vi "LabviewClaDInterface.vi"() -> ()   [LabVIEW 2016]
uses:
  <userlib>/ROS for LabVIEW Software/ROS/Code/SubVIs/_ROSControl.ctl
  <userlib>/ROS for LabVIEW Software/ROS/Code/SubVIs/_ROSDirection.ctl
  <userlib>/ROS for LabVIEW Software/ROS/Code/Console/Servers/ServerSubs/TopicDef.ctl
  <userlib>/ROS for LabVIEW Software/ROS/MessageBuilding/std_msgs/subs/stringScalar.vi
  <userlib>/ROS for LabVIEW Software/ROS/MessageParsing/std_msgs/subs/parse_string_scalar.vi
panel:
  out "Odom Error Out":errorcluster
  out "Scan Error Out":errorcluster
  in  "Stop Subscribing":bool
  out "Husky Pose Plot":cluster{"X":dbl, "Y":dbl}[](graph)=[{"X"=2.1588546690121686, "Y"=0.6824320147682317}]
  out "Laser Scan Plot (in Husky Frame)":cluster{dbl[], dbl[]}(graph)
  out "Husky EKF Odometry":T1={"PoseCovariance"={"Pose"={"Position\n(xyz)"={"x"=2.1588546690121686, "y"=0.6824320147682317, "z"=0.0}, "Orientation\n(Quaternions)"={"x"=0.0, "y"=0.0, "z"=-0.6154075833582808, "w"=0.7882090499005455}}, "Covariance[1,1]"=150.49515067805697}}
  out "2D Pose":cluster{"x":dbl, "y":dbl}={"x"=2.1588546690121686, "y"=0.6824320147682317}
  in  "Update Time (ms)":u32=300
  in  "Clear Plot":bool
  out "Scan Details":T2={"Min. Angle (rad)"=-2.3561899662017822, "Max. Angle (rad)"=2.3561899662017822, "Angle Incr. (rad)"=0.006554075051099062, "Time Inc. (s)"=0.0, "Scan Time (s)"=0.0, "Min. Range (m)"=0.10000000149011612, "Max. Range (m)"=1.0089348943138683e-42}
  in  "Max Odom Pts":dbl=500.0
  out "Robot Velocity":dbl(knob) scale=0.0..10.0
  out "ROS velocity_labview":T3={"topic port"=0, "Node"="", "topic"="", "type"="", "node port"=0, "error "={"status"=FALSE, "code"=0, "source"=""}, "Direction"=enum."Node", "Update (ms)"=1, "FIFO size"=1}
  out "ROS Manuel process":T3={"topic port"=0, "Node"="", "topic"="", "type"="", "node port"=0, "error "={"status"=FALSE, "code"=0, "source"=""}, "Direction"=enum."Node", "Update (ms)"=1, "FIFO size"=1}
  in  "velocity Process Stop":bool
  out "XY Graph":cluster{"X":dbl, "Y":dbl}[](graph)
  in  "Manuel Process Stop":bool
  in  "Message":string
  in  "Autonomous Process Stop":bool
  in  "Right":bool
  in  "Left":bool
  in  "Down":bool
  in  "Up":bool
  in  "Process Stop":bool
  in  "Home":bool
  out "Table  8":bool
  out "Table  7":bool
  out "Table  6":bool
  in  "OK Button":bool
  in  "table 8":bool
  in  "table 7":bool
  out "ROS Autonomous control":T3={"topic port"=0, "Node"="", "topic"="", "type"="", "node port"=0, "error "={"status"=FALSE, "code"=0, "source"=""}, "Direction"=enum."Node", "Update (ms)"=1, "FIFO size"=1}
  in  "table 6":bool
  in  "table 5":bool
  in  "table 4":bool
  in  "table 3":bool
  in  "table2":bool
  in  "table 1":bool
  out "ROS Autonomous indicator Tables":T3={"topic port"=0, "Node"="", "topic"="", "type"="", "node port"=0, "error "={"status"=FALSE, "code"=0, "source"=""}, "Direction"=enum."Node", "Update (ms)"=1, "FIFO size"=1}
  out "Table  5":bool
  out "Table  4":bool
  out "Table  3":bool
  out "Table  2":bool
  out "Table 1":bool
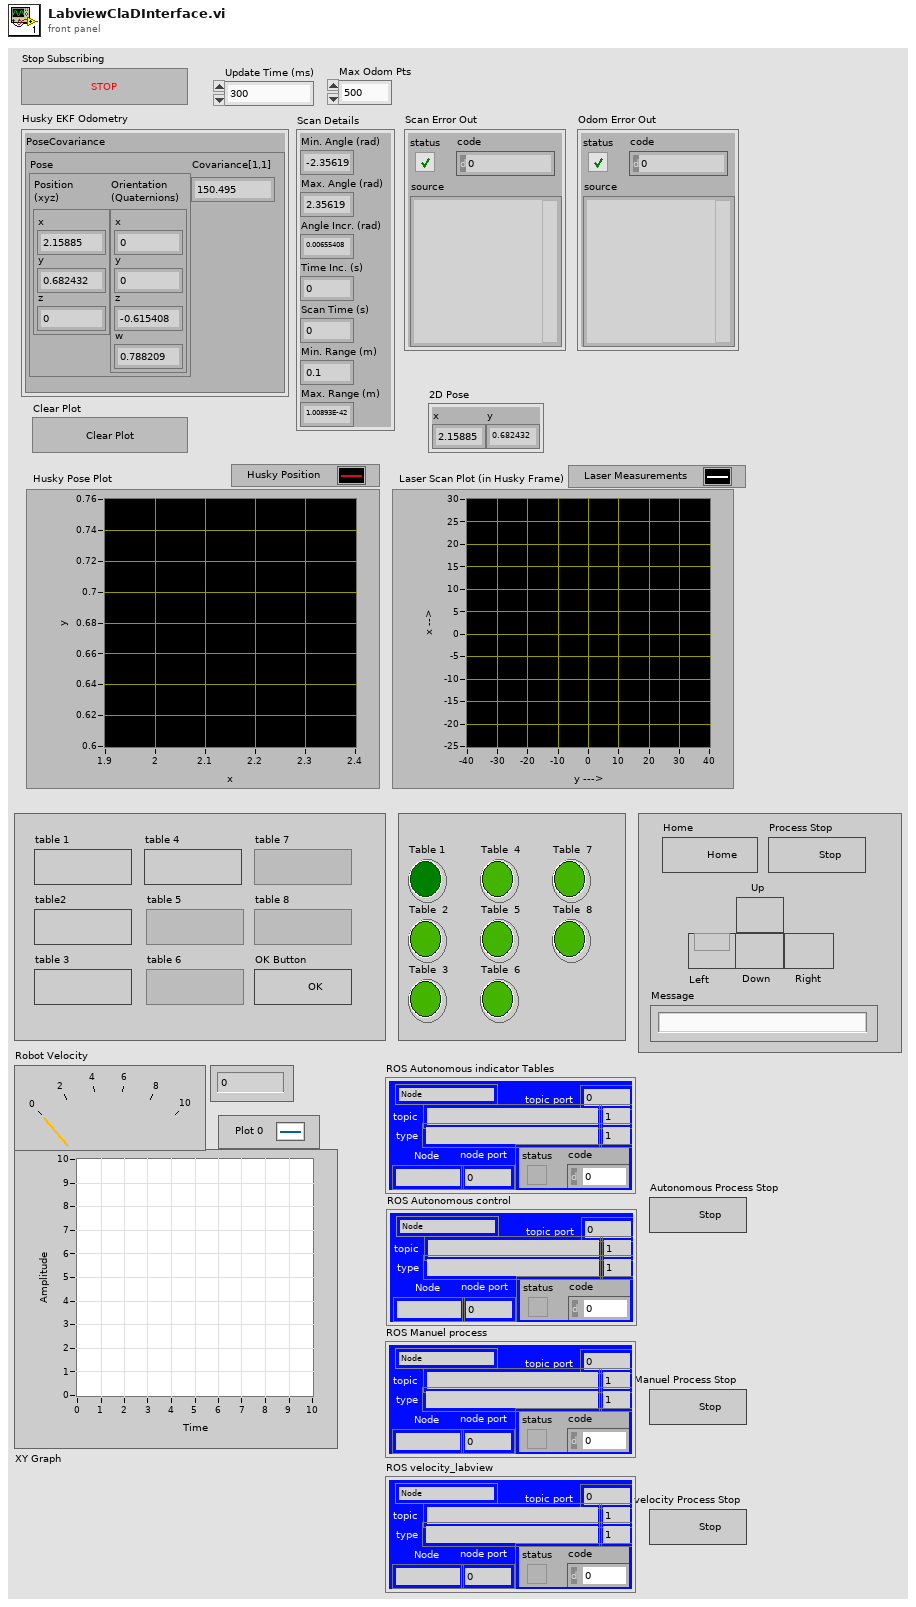
[diagram p1: front panel]
types:
  T1 = cluster{"PoseCovariance":cluster{"Pose":cluster{"Position\n(xyz)":cluster{"x":dbl, "y":dbl, "z":dbl}, "Orientation\n(Quaternions)":cluster{"x":dbl, "y":dbl, "z":dbl, "w":dbl}}, "Covariance[1,1]":dbl}}
  T2 = cluster{"Min. Angle (rad)":dbl, "Max. Angle (rad)":dbl, "Angle Incr. (rad)":dbl, "Time Inc. (s)":dbl, "Scan Time (s)":dbl, "Min. Range (m)":dbl, "Max. Range (m)":dbl}
  T3 = typedef "_ROSControl.ctl" = cluster{"topic port":u16, "Node":string, "topic":string, "type":string, "node port":u16, "error ":errorcluster, "Direction":T4, "Update (ms)":u16, "FIFO size":u16}
  T4 = typedef "_ROSDirection.ctl" = enum16{"Node", "Publisher", "Subscriber", "ServiceClient", "ServiceProvider"}
  T5 = typedef "TopicDef.ctl" = cluster{"Topic":string, "Type":string, "Action":T4, "Update (ms)":u16, "queue size":u16}
  T6 = cluster{"PoseCovariance":cluster{"Pose":cluster{"Point":cluster{"x":dbl, "y":dbl, "z":dbl}, "Quaternion":cluster{"x":dbl, "y":dbl, "z":dbl, "w":dbl}}, "Covariance":dbl}}
  T7 = cluster{"Linear":cluster{"x":dbl, "y":dbl, "z":dbl}, "Angular":cluster{"x":dbl, "y":dbl, "z":dbl}}
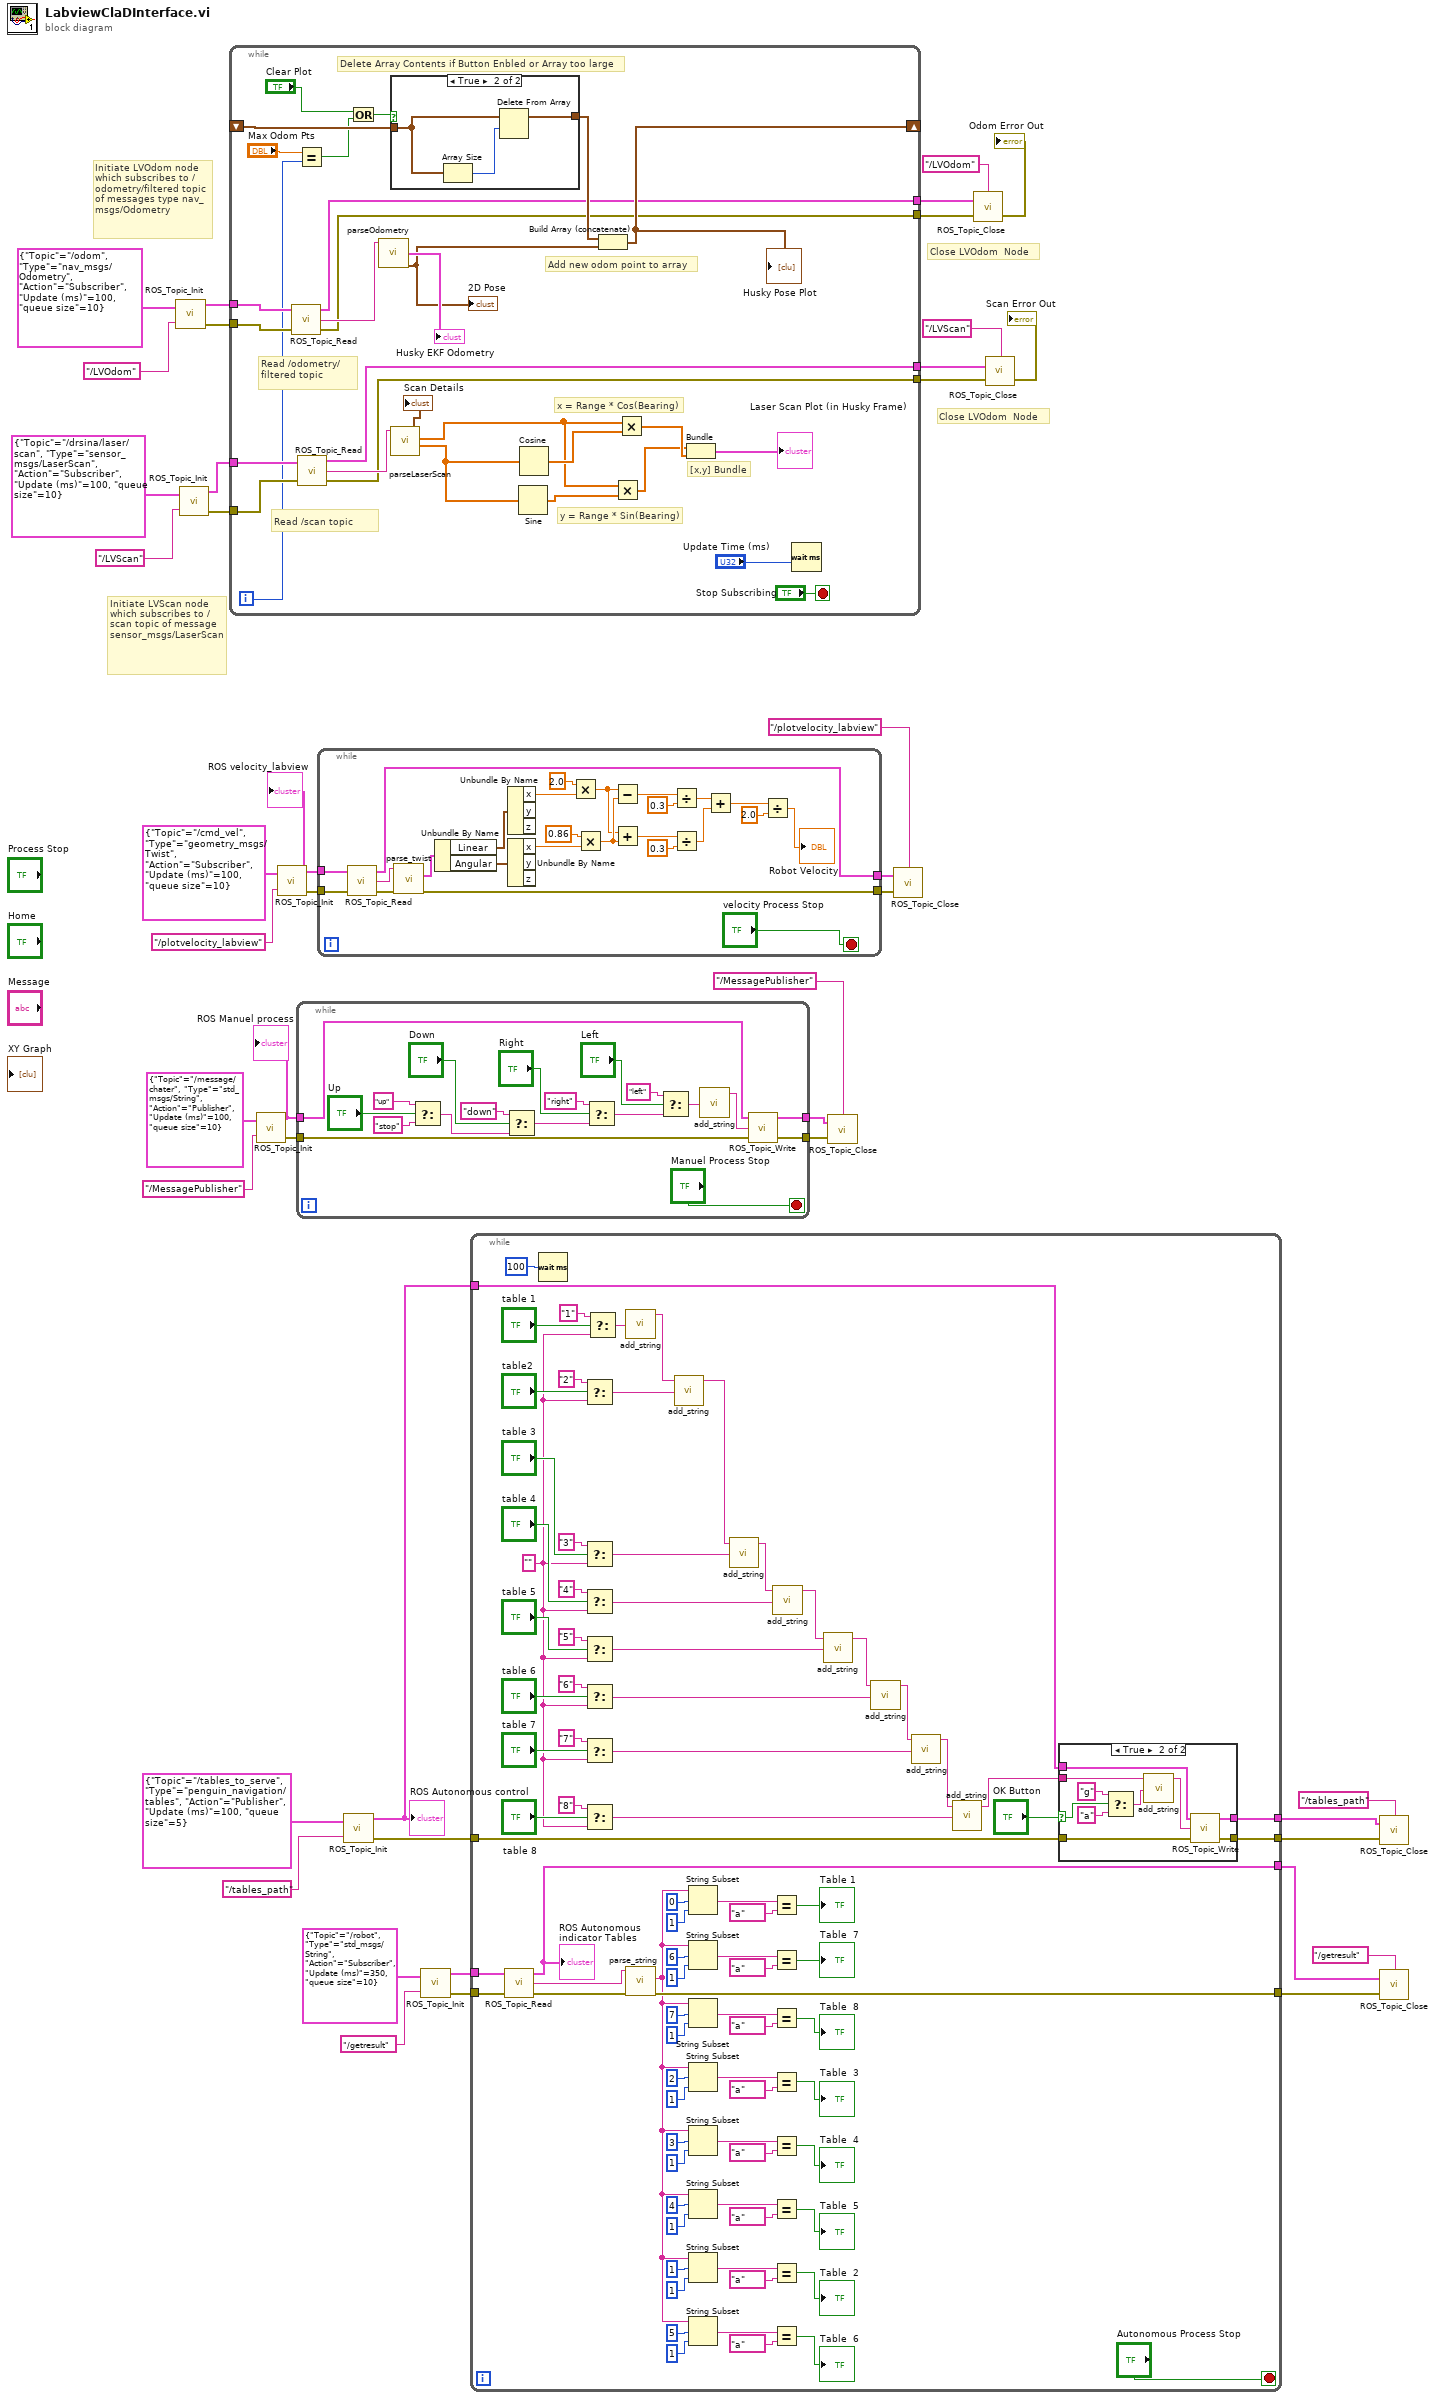
[diagram p0: block diagram]
diagram:
  # "Close LVOdom  Node"
  # "Close LVOdom  Node"
  # "Initiate LVScan node which subscribes to /scan topic of message sensor_msgs/LaserScan"
  # "Initiate LVOdom node which subscribes to /odometry/filtered topic of messages type nav_msgs/Odometry"
  n1 = call <userlib>:"ROS_Topic_Init.vi"("Definitions"=T5 {"Topic"="/odom", "Type"="nav_msgs/Odometry", "Action"=enum."Subscriber", "Update (ms)"=100, "queue size"=10}, "node"="/LVOdom") -> ("ROS out"=w12:T3, "error out"=w11:errorcluster)  [unwired: 1 in]
  n2 = call <userlib>:"ROS_Topic_Init.vi"("Definitions"=T5 {"Topic"="/drsina/laser/scan", "Type"="sensor_msgs/LaserScan", "Action"=enum."Subscriber", "Update (ms)"=100, "queue size"=10}, "node"="/LVScan") -> ("ROS out"=w10:T3, "error out"=w9:errorcluster)  [unwired: 1 in]
  n3 = while {
    shift-right: [w73] -> _
    shift-left: _ -> [w59]
    tunnel: w12 -> [w64]
    tunnel: w11 -> [w63]
    tunnel: w10 -> [w62]
    tunnel: w9 -> [w61]
    tunnel: [w56] -> w8
    tunnel: [w55] -> w7
    tunnel: [w54] -> w5
    tunnel: [w53] -> w3
    i -> [w46]
    stop <- "Stop Subscribing" stop-if-true
    # "Add new odom point to array"
    # "Read /scan topic"
    # "Read /odometry/filtered topic"
    # "Delete Array Contents if Button Enbled or Array too large"
    # "[x,y] Bundle"
    # "y = Range * Sin(Bearing)"
    # "x = Range * Cos(Bearing)"
    n4 = call <userlib>:"ROS_Topic_Read.vi"("error in (no error)"=w63, "ROS in"=w64) -> ("error out"=w53:errorcluster, "Reply"=w72:string, "ROS out"=w55:T3)  [unwired: 1 in]
    n5 = Equal?(x="Max Odom Pts", y=w46) -> (x = y?=w45:bool)
    n6 = call <userlib>:"ROS_Topic_Read.vi"("error in (no error)"=w61, "ROS in"=w62) -> ("error out"=w54:errorcluster, "Reply"=w69:string, "ROS out"=w56:T3)  [unwired: 1 in]
    n7 = Or(x="Clear Plot", y=w45) -> (x .or. y?=w48:bool)
    n8 = call "parseOdometry.vi"("msg in"=w72) -> ("Odometry"=→"Husky EKF Odometry":T6, "Pose 2D"=w70:cluster{"x":dbl, "y":dbl})  [unwired: 3 in, 3 out]
    "2D Pose" <- w70
    n9 = case shown="True" w48 {
      tunnel: [w75 w77] -> w58
      tunnel: w59 -> [w75 w76]
      frame False {
      }
      frame True {
        n10 = Array Size(array=w76) -> (size(s)=w78:i32)
        n11 = Delete From Array "Delete From Array"(array=w76, length=w78) -> (array with subset deleted=w77:cluster{"x":dbl, "y":dbl}[])  [unwired: 1 in, 1 out]
      }
    }
    n12 = call "parseLaserScan.vi"("msg in"=w69) -> ("Bearing Array"=w67:dbl[], "Range Array"=w66:sgl[], "Scan Details"=→"Scan Details":T2)  [unwired: 3 in, 1 out]
    n13 = Sine(x=w67) -> (sin(x)=w65:dbl[])
    n14 = Cosine(x=w67) -> (cos(x)=w68:dbl[])
    n15 = Build Array (concatenate)(w58, w70) -> (w73:cluster{"x":dbl, "y":dbl}[])
    "Husky Pose Plot" <- w73
    n16 = Multiply(x=w66, y=w65) -> (x*y=w51:dbl[])
    n17 = Multiply(x=w66, y=w68) -> (x*y=w52:dbl[])
    n18 = Bundle(w51, w52) -> (→"Laser Scan Plot (in Husky Frame)":cluster{dbl[], dbl[]})  [unwired: 1 in]
    n19 = Wait (ms)(milliseconds to wait="Update Time (ms)") -> ()  [unwired: 1 out]
  }
  n20 = call <userlib>:"ROS_Topic_Init.vi"("Definitions"=T5 {"Topic"="/message/chater", "Type"="std_msgs/String", "Action"=enum."Publisher", "Update (ms)"=100, "queue size"=10}, "node"="/MessagePublisher") -> ("ROS out"=w26:T3, "error out"=w27:errorcluster)  [unwired: 1 in]
  "ROS Manuel process" <- w26
  n21 = call <userlib>:"ROS_Topic_Init.vi"("Definitions"=T5 {"Topic"="/cmd_vel", "Type"="geometry_msgs/Twist", "Action"=enum."Subscriber", "Update (ms)"=100, "queue size"=10}, "node"="/plotvelocity_labview") -> ("ROS out"=w21:T3, "error out"=w20:errorcluster)  [unwired: 1 in]
  "ROS velocity_labview" <- w21
  n22 = while {
    tunnel: w26 -> [w97]
    tunnel: w27 -> [w96]
    tunnel: [w94] -> w28
    tunnel: [w93] -> w29
    stop <- "Manuel Process Stop" stop-if-true
    n23 = Select(t="up", s="Up", f="stop") -> (s? t:f=w90:string)
    n24 = Select(t="down", s="Down", f=w90) -> (s? t:f=w91:string)
    n25 = Select(t="right", s="Right", f=w91) -> (s? t:f=w92:string)
    n26 = Select(t="left", s="Left", f=w92) -> (s? t:f=w84:string)
    n27 = call-poly <userlib>:"add_string.vi"("String"=w84) -> ("msg out"=w95:string)  [unwired: 4 in]
    n28 = call <userlib>:"ROS_Topic_Write.vi"("error in (no error)"=w96, "Msg in"=w95, "ROS in"=w97) -> ("error out"=w93:errorcluster, "ROS out"=w94:T3)  [unwired: 1 in]
  }
  n29 = while {
    tunnel: w21 -> [w121]
    tunnel: w20 -> [w120]
    tunnel: [w117] -> w19
    tunnel: [w116] -> w18
    stop <- "velocity Process Stop" stop-if-true
    n30 = call <userlib>:"ROS_Topic_Read.vi"("error in (no error)"=w120, "ROS in"=w121) -> ("error out"=w118:errorcluster, "Reply"=w119:string, "ROS out"=w117:T3)  [unwired: 1 in]
    n31 = call <userlib>:"parse_twist.vi"("error in"=w118, "msg in"=w119) -> ("error out"=w116:errorcluster, "Twist"=w115:T7)  [unwired: 3 in, 1 out]
    n32 = Unbundle By Name(w115) -> ("Linear"=w114:cluster{"x":dbl, "y":dbl, "z":dbl}, "Angular"=w113:cluster{"x":dbl, "y":dbl, "z":dbl})
    n33 = Unbundle By Name(w114) -> ("x"=w112:dbl)  [unwired: 2 out]
    n34 = Unbundle By Name(w113) -> ("x"=w111:dbl)  [unwired: 2 out]
    n35 = Multiply(x=2.0, y=w112) -> (x*y=w99:dbl)
    n36 = Multiply(x=0.86, y=w111) -> (x*y=w110:dbl)
    n37 = Subtract(x=w99, y=w110) -> (x-y=w108:dbl)
    n38 = Add(x=w99, y=w110) -> (x+y=w109:dbl)
    n39 = Divide(x=w108, y=0.3 ("x")) -> (x/y=w107:dbl)
    n40 = Divide(x=w109, y=0.3 ("x")) -> (x/y=w106:dbl)
    n41 = Add(x=w107, y=w106) -> (x+y=w105:dbl)
    n42 = Divide(x=w105, y=2.0 ("x")) -> (x/y=→"Robot Velocity":dbl)
  }
  n43 = call <userlib>:"ROS_Topic_Init.vi"("Definitions"=T5 {"Topic"="/tables_to_serve", "Type"="penguin_navigation/tables", "Action"=enum."Publisher", "Update (ms)"=100, "queue size"=5}, "node"="/tables_path") -> ("ROS out"=w38:T3, "error out"=w37:errorcluster)  [unwired: 1 in]
  "ROS Autonomous control" <- w38
  n44 = call <userlib>:"ROS_Topic_Init.vi"("Definitions"=T5 {"Topic"="/robot", "Type"="std_msgs/String", "Action"=enum."Subscriber", "Update (ms)"=350, "queue size"=10}, "node"="/getresult") -> ("ROS out"=w34:T3, "error out"=w33:errorcluster)  [unwired: 1 in]
  n45 = while {
    tunnel: w34 -> [w166]
    tunnel: [w164] -> w43
    tunnel: w33 -> [w165]
    tunnel: [w209] -> w42
    tunnel: w38 -> [w159]
    tunnel: w37 -> [w158]
    tunnel: [w157] -> w32
    tunnel: [w156] -> w31
    stop <- "Autonomous Process Stop" stop-if-true
    w151 = "" ("t")
    n46 = call <userlib>:"ROS_Topic_Read.vi"("error in (no error)"=w165, "ROS in"=w166) -> ("error out"=w162:errorcluster, "Reply"=w163:string, "ROS out"=w164:T3)  [unwired: 1 in]
    "ROS Autonomous indicator Tables" <- w164
    n47 = Wait (ms)(milliseconds to wait=u32 100) -> ()  [unwired: 1 out]
    n48 = Select(t="2", s="table2", f=w151) -> (s? t:f=w204:string)
    n49 = Select(t="3", s="table 3", f=w151) -> (s? t:f=w205:string)
    n50 = Select(t="4", s="table 4", f=w151) -> (s? t:f=w206:string)
    n51 = Select(t="5", s="table 5", f=w151) -> (s? t:f=w207:string)
    n52 = Select(t="6", s="table 6", f=w151) -> (s? t:f=w147:string)
    n53 = Select(t="7", s="table 7", f=w151) -> (s? t:f=w146:string)
    n54 = Select(t="8", s="table 8", f=w151) -> (s? t:f=w145:string)
    n55 = Select(t="1", s="table 1", f=w151) -> (s? t:f=w161:string)
    n56 = call-poly <userlib>:"add_string.vi"("String"=w161) -> ("msg out"=w160:string)  [unwired: 4 in]
    n57 = call-poly <userlib>:"parse_string.vi"("error in"=w162, "msg in"=w163) -> ("error out"=w209:errorcluster, "string"=w123:string)  [unwired: 3 in, 1 out]
    n58 = call-poly <userlib>:"add_string.vi"("String"=w204, "msg in"=w160) -> ("msg out"=w203:string)  [unwired: 3 in]
    n59 = String Subset(string=w123, offset (0)=0, length (rest)=1 ("offset (0)")) -> (substring=w181:string)
    n60 = String Subset(string=w123, offset (0)=6, length (rest)=1 ("offset (0)")) -> (substring=w132:string)
    n61 = String Subset(string=w123, offset (0)=7, length (rest)=1 ("offset (0)")) -> (substring=w126:string)
    n62 = String Subset(string=w123, offset (0)=2, length (rest)=1 ("offset (0)")) -> (substring=w179:string)
    n63 = String Subset(string=w123, offset (0)=3, length (rest)=1 ("offset (0)")) -> (substring=w178:string)
    n64 = String Subset(string=w123, offset (0)=4, length (rest)=1 ("offset (0)")) -> (substring=w177:string)
    n65 = String Subset(string=w123, offset (0)=1, length (rest)=1 ("offset (0)")) -> (substring=w180:string)
    n66 = String Subset(string=w123, offset (0)=5, length (rest)=1 ("offset (0)")) -> (substring=w136:string)
    n67 = call-poly <userlib>:"add_string.vi"("String"=w205, "msg in"=w203) -> ("msg out"=w202:string)  [unwired: 3 in]
    n68 = Equal?(x=w181, y="a") -> (x = y?=→"Table 1":bool)
    n69 = Equal?(x=w132, y="a") -> (x = y?=→"Table  7":bool)
    n70 = Equal?(x=w126, y="a") -> (x = y?=→"Table  8":bool)
    n71 = Equal?(x=w179, y="a") -> (x = y?=→"Table  3":bool)
    n72 = Equal?(x=w178, y="a") -> (x = y?=→"Table  4":bool)
    n73 = Equal?(x=w177, y="a") -> (x = y?=→"Table  5":bool)
    n74 = Equal?(x=w180, y="a") -> (x = y?=→"Table  2":bool)
    n75 = Equal?(x=w136, y="a") -> (x = y?=→"Table  6":bool)
    n76 = call-poly <userlib>:"add_string.vi"("String"=w206, "msg in"=w202) -> ("msg out"=w208:string)  [unwired: 3 in]
    n77 = call-poly <userlib>:"add_string.vi"("String"=w207, "msg in"=w208) -> ("msg out"=w144:string)  [unwired: 3 in]
    n78 = call-poly <userlib>:"add_string.vi"("String"=w147, "msg in"=w144) -> ("msg out"=w143:string)  [unwired: 3 in]
    n79 = call-poly <userlib>:"add_string.vi"("String"=w146, "msg in"=w143) -> ("msg out"=w142:string)  [unwired: 3 in]
    n80 = call-poly <userlib>:"add_string.vi"("String"=w145, "msg in"=w142) -> ("msg out"=w141:string)  [unwired: 3 in]
    n81 = case shown="True" "OK Button" {
      selector: "OK Button" -> [_ w215]
      tunnel: w141 -> [_ w217]
      tunnel: w159 -> [_ w213]
      tunnel: w158 -> [_ w212]
      tunnel: [_ w211] -> w157
      tunnel: [_ w210] -> w156
      frame False {
      }
      frame True {
        n82 = Select(t="g", s=w215, f="a") -> (s? t:f=w216:string)
        n83 = call-poly <userlib>:"add_string.vi"("String"=w216, "msg in"=w217) -> ("msg out"=w214:string)  [unwired: 3 in]
        n84 = call <userlib>:"ROS_Topic_Write.vi"("error in (no error)"=w212, "Msg in"=w214, "ROS in"=w213) -> ("error out"=w211:errorcluster, "ROS out"=w210:T3)  [unwired: 1 in]
      }
    }
  }
  n85 = call <userlib>:"ROS_Topic_Close.vi"("error in"=w29, "ROS in"=w28, "node"="/MessagePublisher") -> ()  [unwired: 1 in, 1 out]
  n86 = call <userlib>:"ROS_Topic_Close.vi"("error in"=w18, "ROS in"=w19, "node"="/plotvelocity_labview") -> ()  [unwired: 1 in, 1 out]
  n87 = call <userlib>:"ROS_Topic_Close.vi"("error in"=w3, "ROS in"=w7, "node"="/LVOdom") -> ("error out"=→"Odom Error Out":errorcluster)  [unwired: 1 in]
  n88 = call <userlib>:"ROS_Topic_Close.vi"("error in"=w5, "ROS in"=w8, "node"="/LVScan") -> ("error out"=→"Scan Error Out":errorcluster)  [unwired: 1 in]
  n89 = call <userlib>:"ROS_Topic_Close.vi"("error in"=w32, "ROS in"=w31, "node"="/tables_path") -> ()  [unwired: 1 in, 1 out]
  n90 = call <userlib>:"ROS_Topic_Close.vi"("error in"=w42, "ROS in"=w43, "node"="/getresult") -> ()  [unwired: 1 in, 1 out]
